vi "Set Delay Generator.vi"(9 "typ":i32, 10 "address":i16, 11 "board":i32) -> (3 "function return":u32)   [LabVIEW 2018, in "AndorSDK.lvlib"]
doc: "EXPNETTYPE unsigned int WINAPI SetDelayGenerator(int board, short address, int typ);"
uses:
  AndorSDK.lvlib
  ATMCD32D.dll
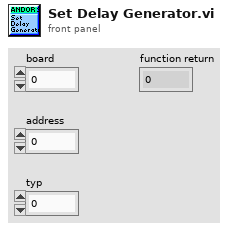
[diagram p1: front panel]
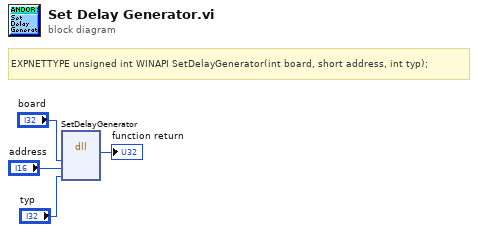
[diagram p0: block diagram]
diagram:
  # "EXPNETTYPE unsigned int WINAPI SetDelayGenerator(int board, short address, int typ);"
  n1 = dll-call lib="PTH2babs E\nPersönliches02 - Arbeit03-HiwijobsLabviewCodelibANDOR\tAndor SDK\nATMCD32D.*" fn="SetDelayGenerator"("board"="board", "address"="address", "typ"="typ") -> (→"function return":u32)  [unwired: 6 in, 2 out]
